vi "Teperature and FIeld Sweep_1022D.vi"() -> ()   [LabVIEW 2022 SP3]
uses:
  <vilib>/Analysis/baseanly.llb/Mean (DBL).vi
  <vilib>/Utility/file.llb/Write Delimited Spreadsheet (DBL).vi
  <vilib>/Analysis/NI_AALBase.lvlib
panel:
  in  "?":bool
  out "Temperature Status":i32(ring) items=["TemperatureUnknown"=0, "Stable"=1, "Tracking"=2, "Near"=5, "Chasing"=6, "Filling"=7, "Standby"=10, "Disabled"=13, "ImpedanceNotFunction"=14, "TempFailure"=15]
  out "Field Status":i32(ring) items=["MagnetUnknown"=0, "StablePersistent"=1, "WarmingSwitch"=2, "CoolingSwitch"=3, "StableDriven"=4, "Iterating"=5, "Charging"=6, "Discharging"=7, "CurrentError"=8, "MagnetFailure"=15]
  out "Field":dbl
  out "Temperature":dbl
  in  "Initialize":bool
  in  "System Stablization (s)":dbl=0.1 format="%#_13g"
  in  "Low Value (Oe)":dbl=-30000.0
  in  "High Value (Oe)":dbl=30000.0
  in  "Sweep Field Approach":i32(ring) items=["Linear", "NoOvershoot", "Oscillate"]
  in  "Sweep F Rate (Oe/s)":dbl=200.0 format="%#_13g"
  in  "Sweep F mode":i32(ring) items=["Persistent", "Driven"]
  in  "Set Fixed T":dbl=2.0
  in  "Fixed Temperature Approach":i32(ring)=1 items=["FastSettle", "NoOvershoot"]
  in  "FIxed T  Rate (K/min)":dbl=20.0
  out "PhaseA-F":cluster{dbl[], dbl[]}(graph)
  out "RA-F":cluster{dbl[], dbl[]}(graph)
  out "Phaseh1B-F":cluster{dbl[], dbl[]}(graph)
  out "Rh1B-F":cluster{dbl[], dbl[]}(graph)
  out "phase B 2":dbl
  in  "Phase B 2":u16(ring)=3 items=["X", "Y", "R", "Theta", "Frequency", "Noise", "Xh1", "Yh1", "Rh1", "Theta h1", "Xh2", "Yh2", "Rh2", "Theta h2"]
  out "phase A 2":dbl
  in  "Phase A 2":u16(ring)=3 items=["X", "Y", "R", "Theta", "Frequency", "Noise", "Xh1", "Yh1", "Rh1", "Theta h1", "Xh2", "Yh2", "Rh2", "Theta h2"]
  out "para1 Measurement (mV) 2":dbl=1.49013e-07
  in  "F Clear Plot A":bool
  in  "Parameter A 2":u16(ring)=2 items=["X", "Y", "R", "Theta", "Frequency", "Noise", "Xh1", "Yh1", "Rh1", "Theta h1", "Xh2", "Yh2", "Rh2", "Theta h2"]
  out "para2 Measurement (uV) 2":dbl=1.49013e-07
  in  "F Clear Plot B":bool
  in  "Parameter B 2":u16(ring)=2 items=["X", "Y", "R", "Theta", "Frequency", "Noise", "Xh1", "Yh1", "Rh1", "Theta h1", "Xh2", "Yh2", "Rh2", "Theta h2"]
  out "Field Setting":dbl format="%#_13g"
  out "Fixed Temperature":dbl
  out "Measured Field":dbl
  out "Field Status":i32(ring) items=["MagnetUnknown"=0, "StablePersistent"=1, "WarmingSwitch"=2, "CoolingSwitch"=3, "StableDriven"=4, "Iterating"=5, "Charging"=6, "Discharging"=7, "CurrentError"=8, "MagnetFailure"=15]
  out "Temperature Status":i32(ring) items=["TemperatureUnknown"=0, "Stable"=1, "Tracking"=2, "Near"=5, "Chasing"=6, "Filling"=7, "Standby"=10, "Disabled"=13, "ImpedanceNotFunction"=14, "TempFailure"=15]
  out "Measuring F":bool
  in  "Step(Oe)":i32=2000
  out "F loop run":i32
  out "Temperature Status":i32(ring) items=["TemperatureUnknown"=0, "Stable"=1, "Tracking"=2, "Near"=5, "Chasing"=6, "Filling"=7, "Standby"=10, "Disabled"=13, "ImpedanceNotFunction"=14, "TempFailure"=15]
  out "Field Status":i32(ring) items=["MagnetUnknown"=0, "StablePersistent"=1, "WarmingSwitch"=2, "CoolingSwitch"=3, "StableDriven"=4, "Iterating"=5, "Charging"=6, "Discharging"=7, "CurrentError"=8, "MagnetFailure"=15]
  out "Fixed Field":dbl
  out "Measured Temperature":dbl
  in  "Delay(T/F)":dbl=3000.0
  in  "Set FIxed F (Oe)":dbl format="%#_13g"
  in  "Fixed Field Approach":i32(ring) items=["Linear", "NoOvershoot", "Oscillate"]
  in  "FIxed F Rate (Oe/s)":dbl=100.0 format="%#_13g"
  in  "Fixed F mode":i32(ring) items=["Persistent", "Driven"]
  in  "Sweep Temperature Approach":i32(ring)=1 items=["FastSettle", "NoOvershoot"]
  in  "Sweep T  Rate (K/min)":dbl=10.0
  in  "Sweep T/F":bool=TRUE
  in  "Remote":bool=TRUE
  in  "IP Address":string="169.254.170.239"
  out "Measuring T":bool
  in  "A Sine Output Amplitude (V)":sgl=0.1
  in  "path (folder + filename)":string="G:\\My Drive\\Opticool\\Measurement\\TF dependence\\TaI23_A67_B68_267Hz_20kOhm_0.1V"
  in  "LOCKIN address":refnum<visa-resource-name>="COM4"
  out "PhaseA-T":cluster{dbl[], dbl[]}(graph)
  out "RA-T":cluster{dbl[], dbl[]}(graph)
  out "Phaseh1-T":cluster{dbl[], dbl[]}(graph)
  out "Rh1B-T":cluster{dbl[], dbl[]}(graph)
  out "phase B":dbl
  in  "Phase B":u16(ring)=9 items=["X", "Y", "R", "Theta", "Frequency", "Noise", "Xh1", "Yh1", "Rh1", "Theta h1", "Xh2", "Yh2", "Rh2", "Theta h2"]
  out "phase A":dbl
  in  "Phase A":u16(ring)=3 items=["X", "Y", "R", "Theta", "Frequency", "Noise", "Xh1", "Yh1", "Rh1", "Theta h1", "Xh2", "Yh2", "Rh2", "Theta h2"]
  out "para1 Measurement (mV)":dbl=1.49013e-07
  in  "T Clear Plot A":bool
  in  "Parameter A":u16(ring)=2 items=["X", "Y", "R", "Theta", "Frequency", "Noise", "Xh1", "Yh1", "Rh1", "Theta h1", "Xh2", "Yh2", "Rh2", "Theta h2"]
  out "para2 Measurement (uV)":dbl=1.49013e-07
  in  "T Clear Plot B":bool
  in  "Parameter B":u16(ring)=8 items=["X", "Y", "R", "Theta", "Frequency", "Noise", "Xh1", "Yh1", "Rh1", "Theta h1", "Xh2", "Yh2", "Rh2", "Theta h2"]
  out "Temperature Setting":dbl format="%#_13g"
  in  "Save data or not":bool=TRUE
  in  "Step(K)":i32=10
  out "T loop run":i32
  in  "B frequency":dbl=267.7 format="%#_13g"
  in  "B Input Connection (0: Single-Ended)":u16(ring)=1 items=["Single-Ended Voltage", "Differential Voltage", "1 MOhm Current Gain", "100 MOhm Current Gain"]
  in  "B harmonic 1":u8=2
  in  "B harmonic 2":u8=3
  in  "B reference Manual Phase":dbl=-59.75
  in  "auto phase B":bool=TRUE
  in  "B Sample time (s)":dbl=0.001 min=0.001 max=100.0 step=0.001
  in  "B Sensitivity":u16(ring)=20 items=["1 nV/fA", "2 nV/fA", "5 nV/fA", "10 nV/fA", "20 nV/fA", "50 nV/fA", "100 nV/fA", "200 nV/fA", "500 nV/fA", "1 uV/pA", "2 uV/pA", "5 uV/pA", "10 uV/pA", "20 uV/pA", "50 uV/pA", "100 uV/pA", "200 uV/pA", "500 uV/pA", "1 mV/nA", "2 mV/nA", "5 mV/nA", "10 mV/nA", "20 mV/nA", "50 mV/nA", "100 mV/nA", "200 mV/nA", "500 mV/nA", "1 V/uA"]
  in  "Enable Sync Filter B (open when f<200Hz)":bool
  in  "B Time Constant":u8(ring)=9 items=["10 us", "30 us", "100 us", "300 us", "1 ms", "3 ms", "10 ms", "30 ms", "100 ms", "300 ms", "1 s", "3 s", "10 s", "30 s", "100 s", "300 s", "1 ks", "3 ks"]
  in  "B Reference Source":u8(ring)=3 items=["External", "Internal", "Internal Sweep", "Channel-A"]
  in  "B Low Pass Filter Slope":u8(ring)=2 items=["6 dB/oct", "12 dB/oct", "18 db/oct", "24 dB/oct"]
  in  "A frequency":dbl=267.7 format="%#_13g"
  in  "A Input Connection (0: Single-Ended)":u16(ring)=1 items=["Single-Ended Voltage", "Differential Voltage", "1 MOhm Current Gain", "100 MOhm Current Gain"]
  in  "A harmonic 1":u8=2
  in  "A harmonic 2":u8=3
  in  "A reference Manual Phase":dbl=-59.75
  in  "auto phase A":bool=TRUE
  in  "A Reference Source":u8(ring)=1 items=["External", "Internal", "Internal Sweep"]
  in  "A Sample time (s)":dbl=0.001 min=0.001 max=100.0 step=0.001
  in  "A Time Constant":u8(ring)=9 items=["10 us", "30 us", "100 us", "300 us", "1 ms", "3 ms", "10 ms", "30 ms", "100 ms", "300 ms", "1 s", "3 s", "10 s", "30 s", "100 s", "300 s", "1 ks", "3 ks"]
  in  "Enable Sync Filter A (open when f<200Hz)":bool
  in  "A Sensitivity":u16(ring)=20 items=["1 nV/fA", "2 nV/fA", "5 nV/fA", "10 nV/fA", "20 nV/fA", "50 nV/fA", "100 nV/fA", "200 nV/fA", "500 nV/fA", "1 uV/pA", "2 uV/pA", "5 uV/pA", "10 uV/pA", "20 uV/pA", "50 uV/pA", "100 uV/pA", "200 uV/pA", "500 uV/pA", "1 mV/nA", "2 mV/nA", "5 mV/nA", "10 mV/nA", "20 mV/nA", "50 mV/nA", "100 mV/nA", "200 mV/nA", "500 mV/nA", "1 V/uA"]
  in  "A Low Pass Filter Slope":u8(ring)=2 items=["6 dB/oct", "12 dB/oct", "18 db/oct", "24 dB/oct"]
  in  "stabilization(S)":dbl=0.1 format="%#_13g"
  in  "High Value (K)":dbl=300.0
  in  "Low Value (K)":dbl=2.0
  in  "loop #":i32=1
  # "Statue"
  # "Lock-in Setting"
  # "Channel A"
  # "Channel B"
  # "Sweep F Mesurement"
  # "Temprature and Field Setting"
  # "Sweep T Mesurement"
  # "Sweep F"
  # "Sweep T"
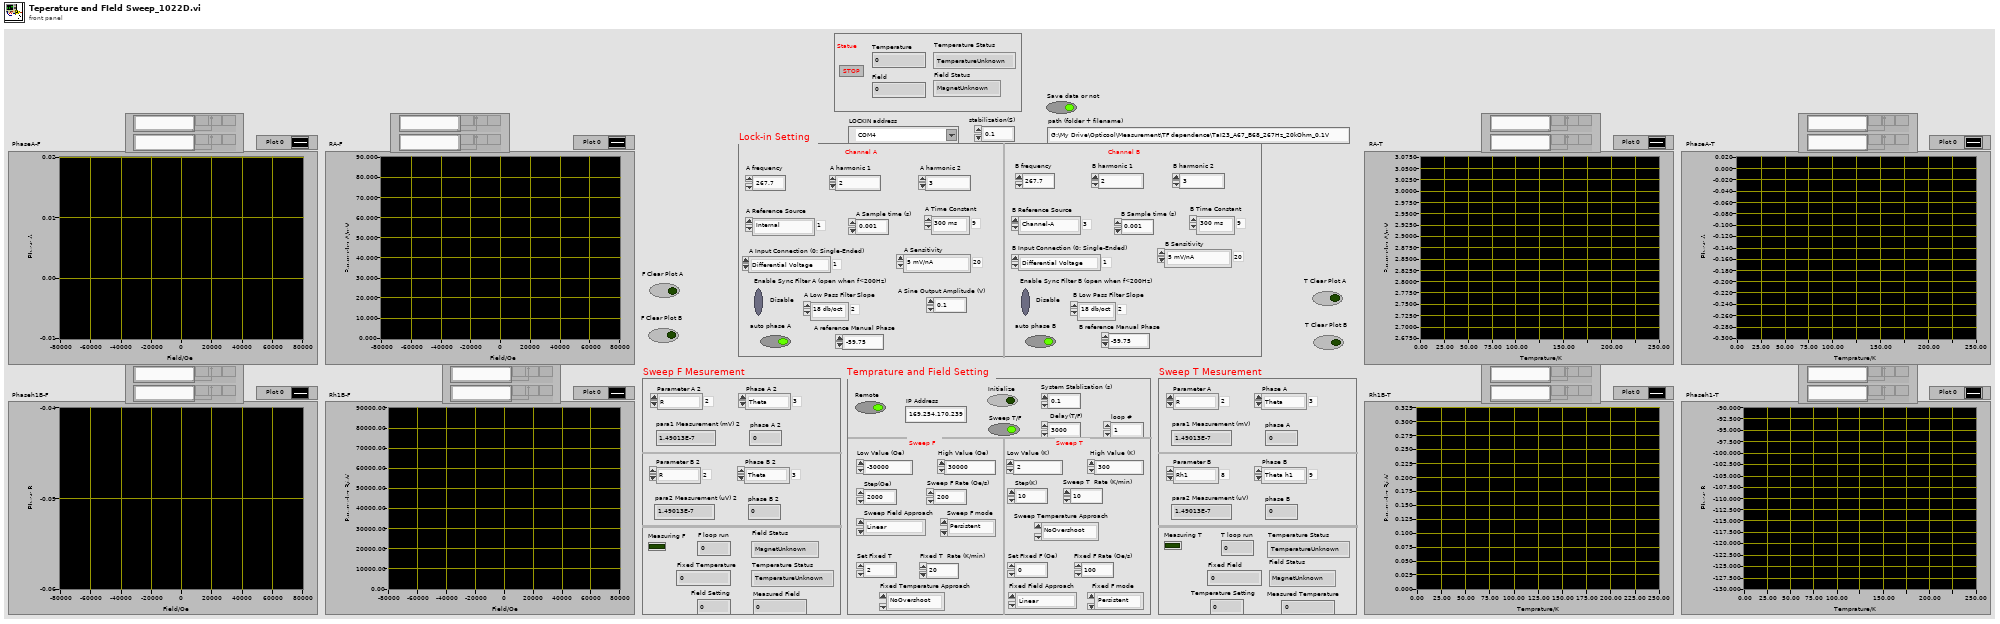
[diagram p1: front panel]
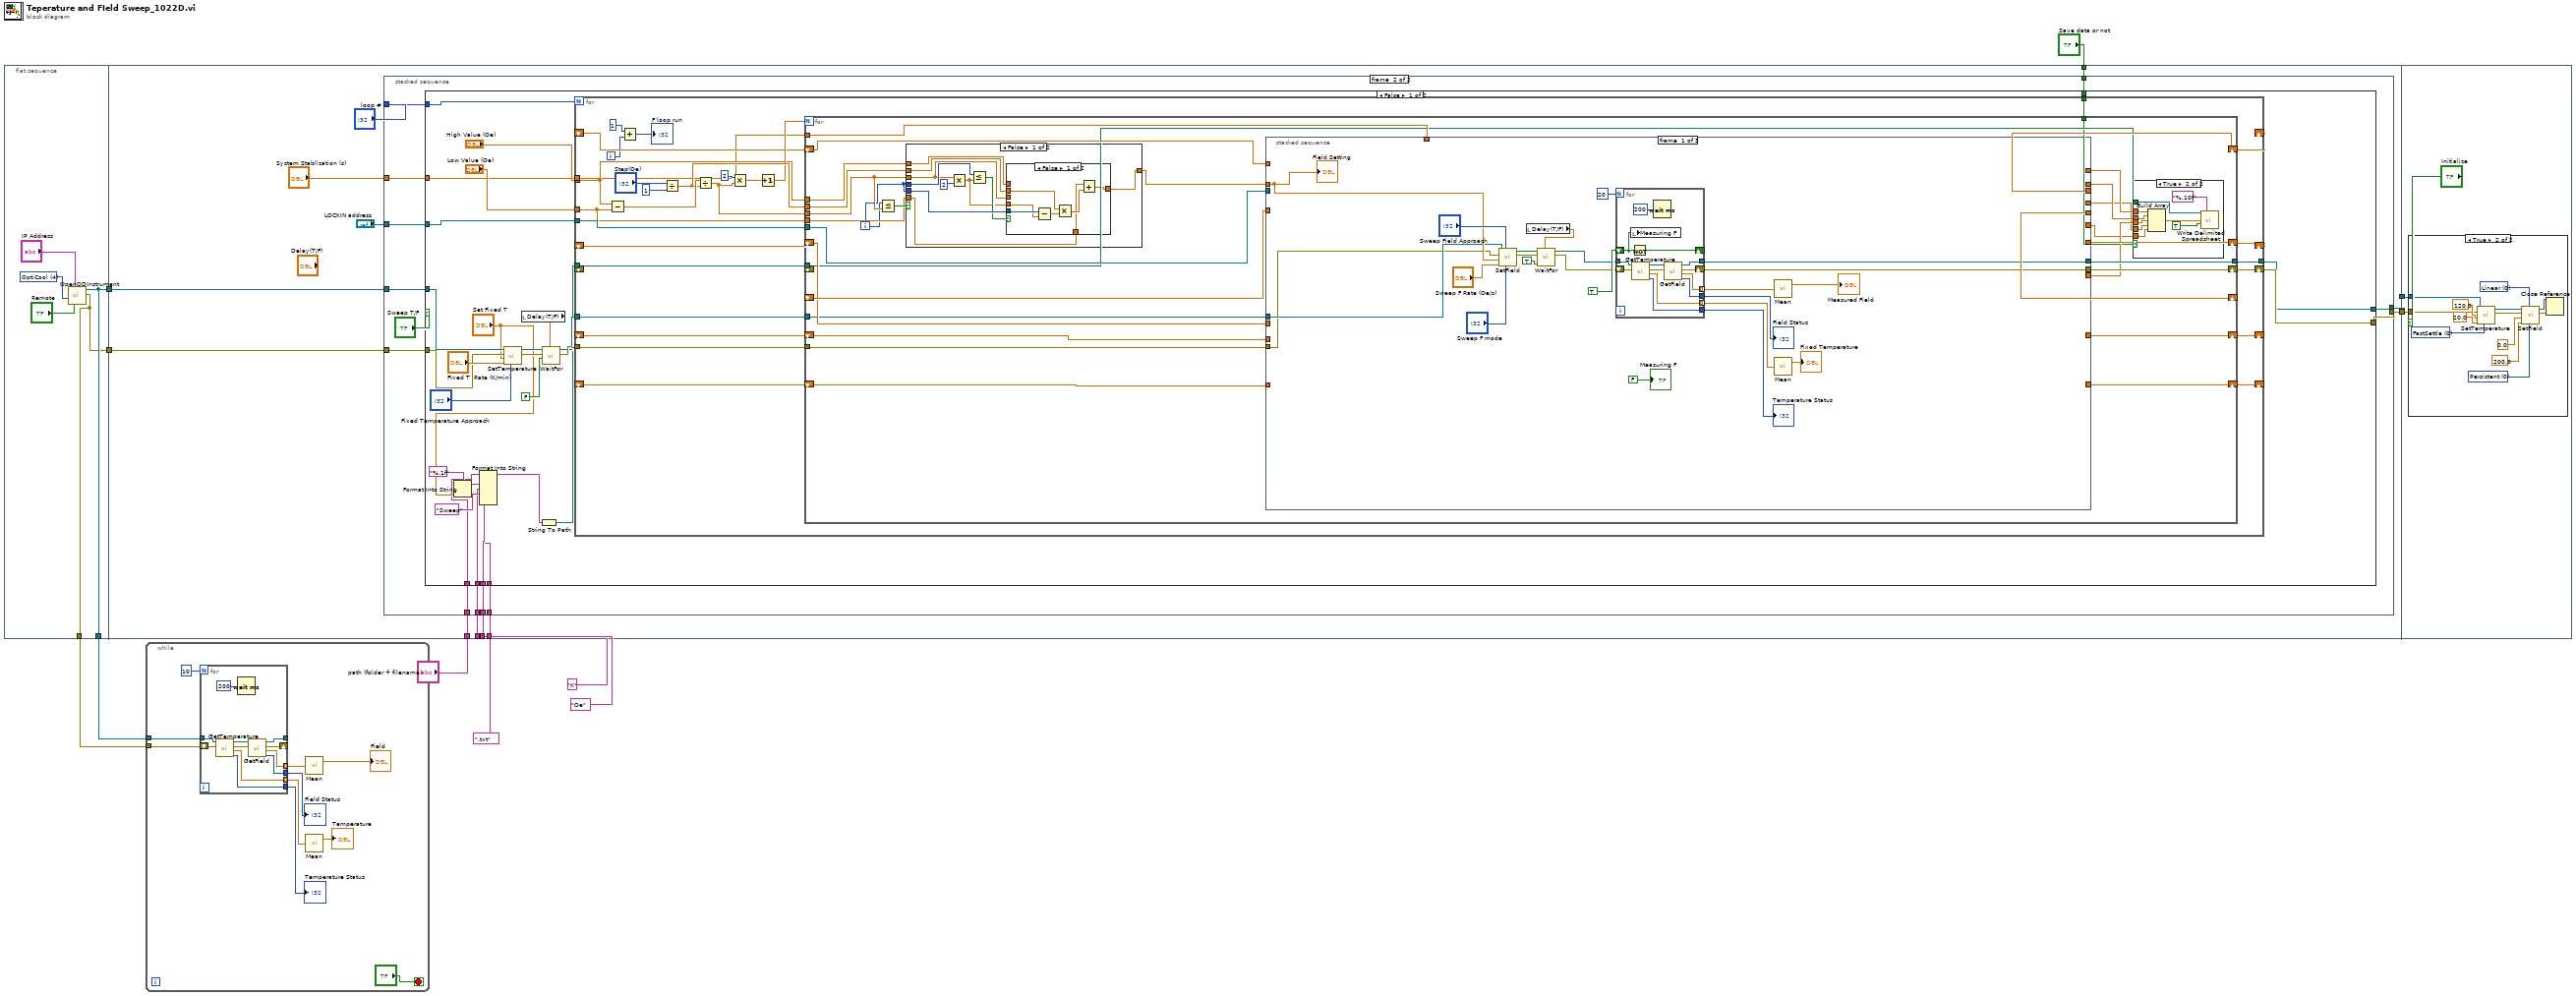
[diagram p0: block diagram]
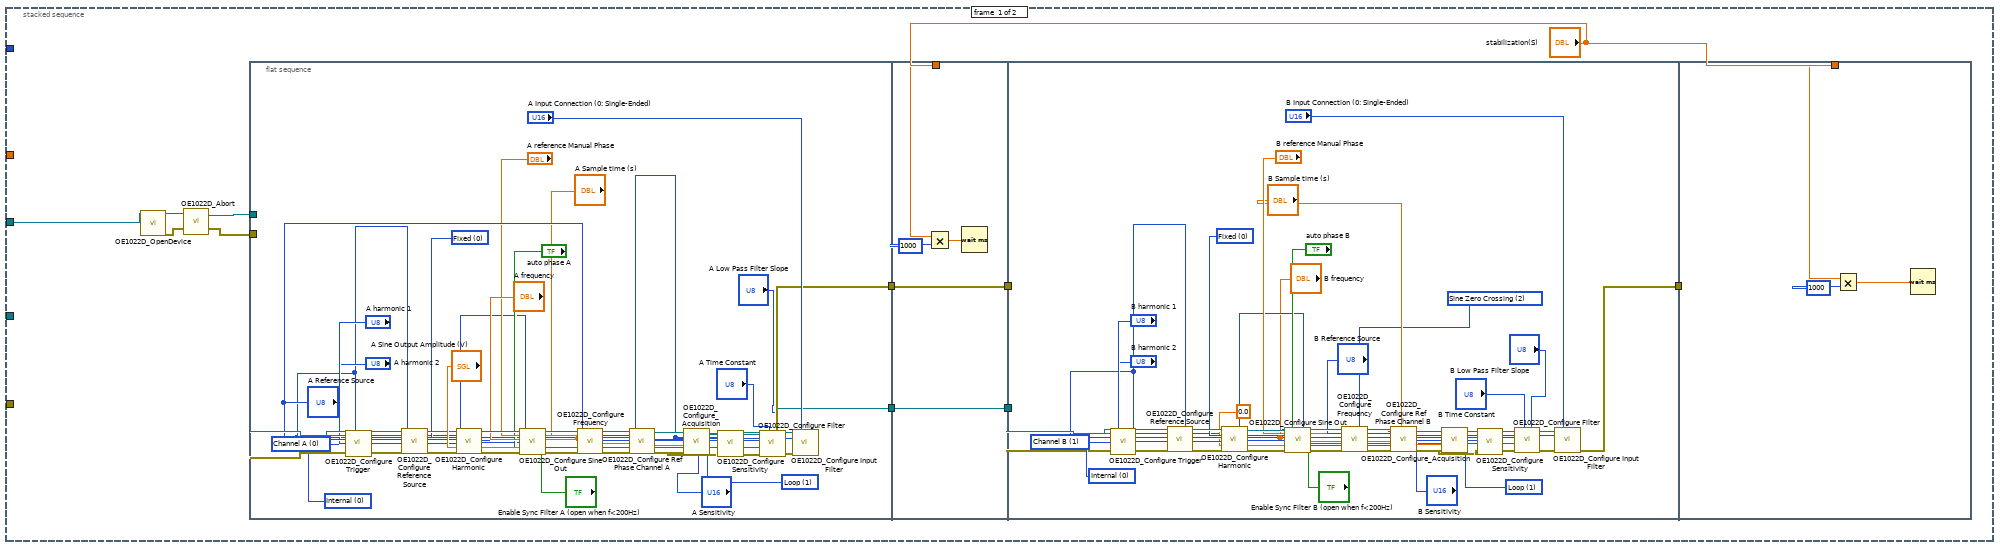
[diagram p2: hidden frame]
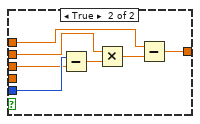
[diagram p4: hidden frame]
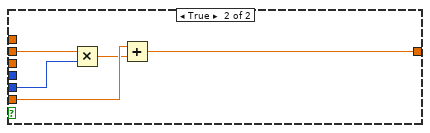
[diagram p5: hidden frame]
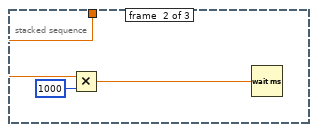
[diagram p6: hidden frame]
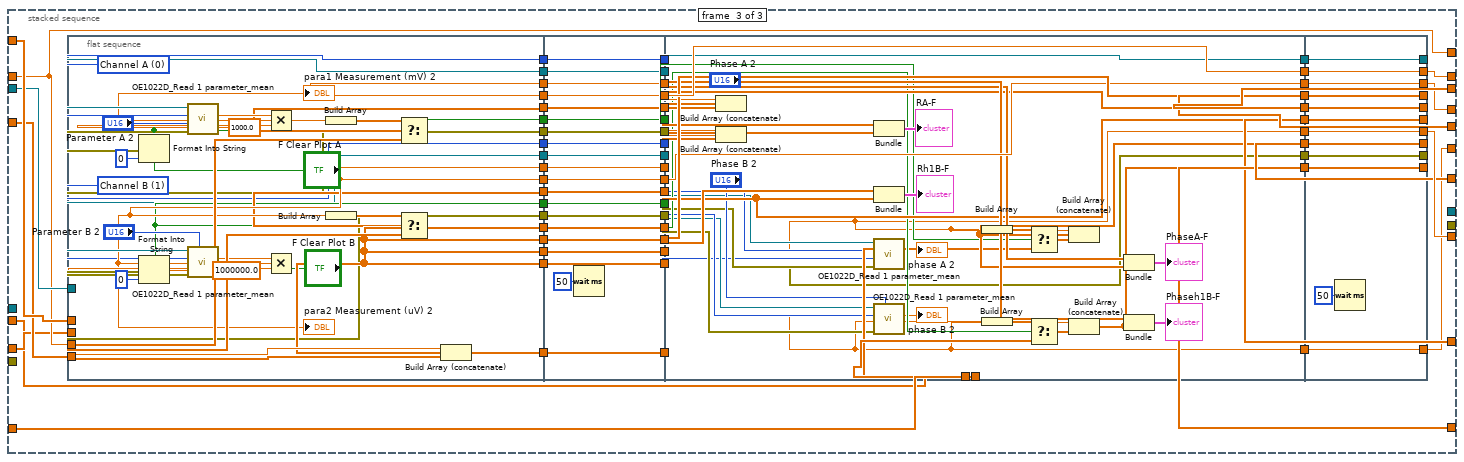
[diagram p7: hidden frame]
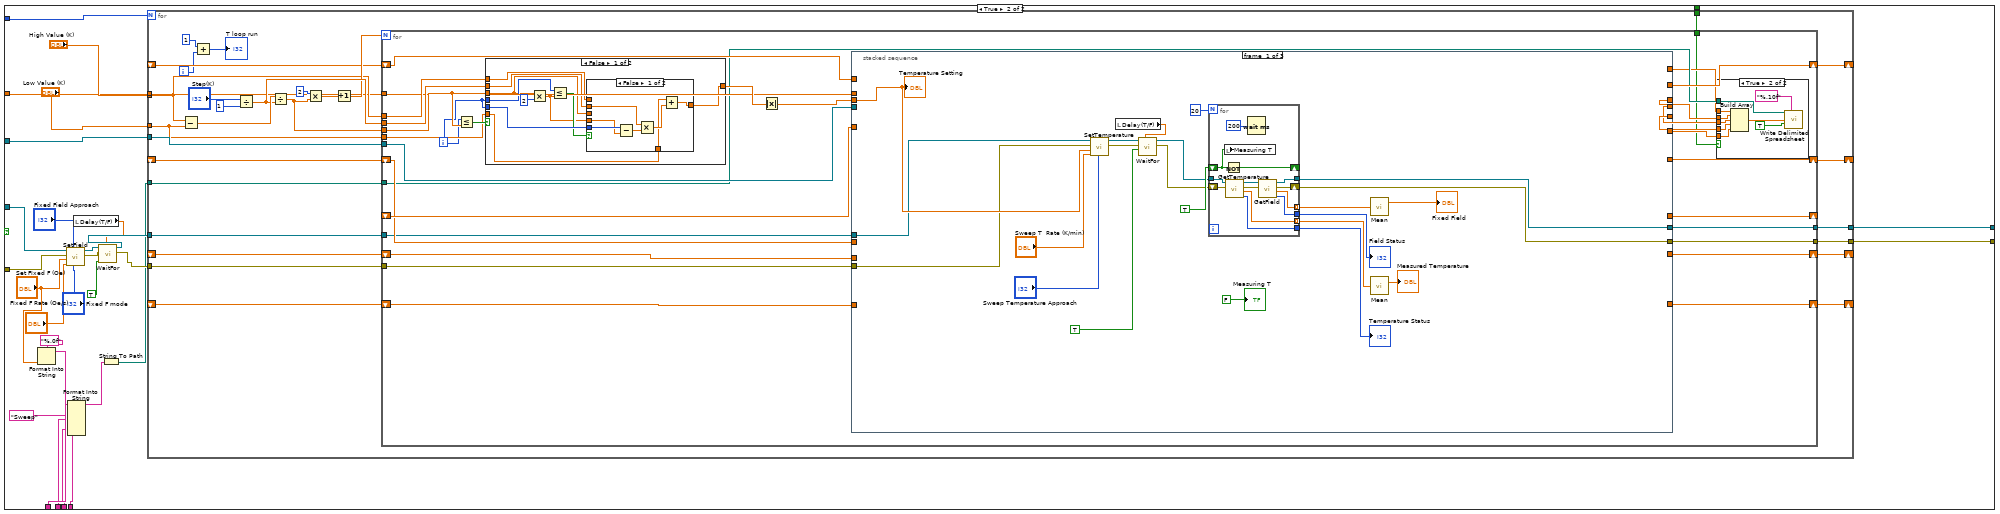
[diagram p8: hidden frame]
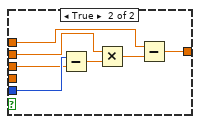
[diagram p10: hidden frame]
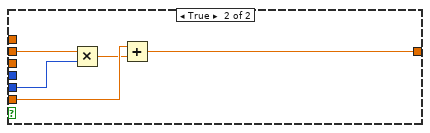
[diagram p11: hidden frame]
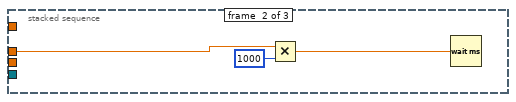
[diagram p12: hidden frame]
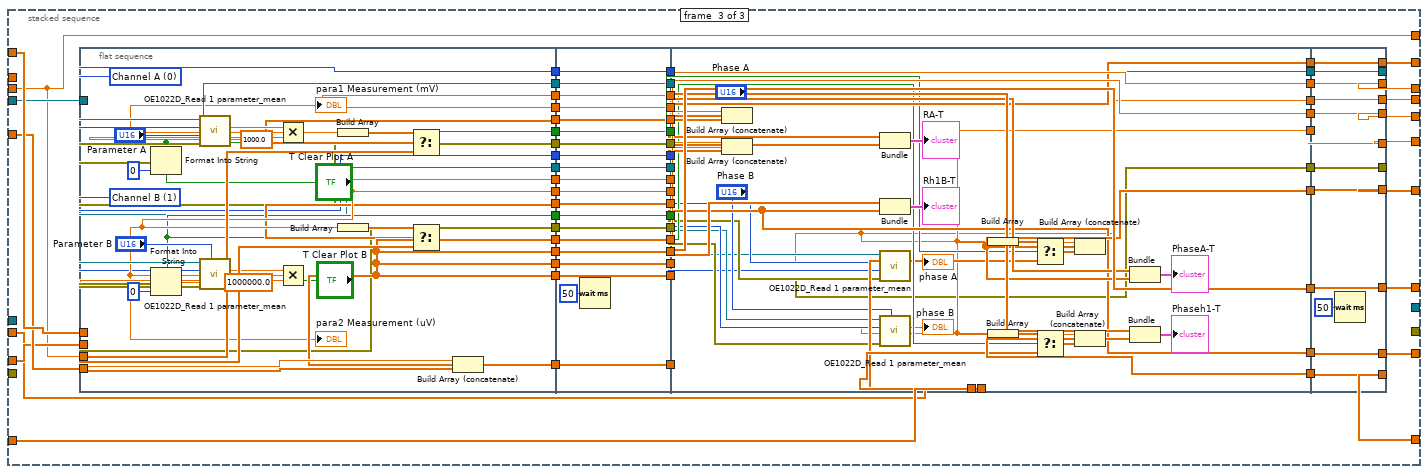
[diagram p13: hidden frame]
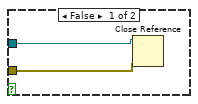
[diagram p14: hidden frame]
diagram:
  n1 = flat-sequence {
    tunnel: [w13] -> w11
    tunnel: [w12] -> w10
    tunnel: [w13] -> w3
    tunnel: [w12] -> w2
    tunnel: w11 -> [w26]
    tunnel: w10 -> [w25]
    tunnel: "path (folder + filename)" -> [w24]
    tunnel: "Oe" -> [w23]
    tunnel: "K" -> [w22]
    tunnel: ".txt" -> [w21]
    tunnel: [w19] -> w5
    tunnel: [w18] -> w4
    tunnel: "Save data or not" -> [w17]
    tunnel: w5 -> [w800]
    tunnel: w4 -> [w799]
    frame #0 {
      w14 = 4 items=["PPMS", "VersaLab", "DynaCool", "SVSM", "OptiCool"] ("InstrumentType")
      n2 = call "OpenQDInstrument.vi"("Remote"="Remote", "IP Address"="IP Address", "InstrumentType"=w14) -> ("error out"=w12:errorcluster, "Instrument Ref"=w13:refnum<k24>)  [unwired: 5 in]
    }
    frame #1 {
      n3 = stacked-sequence {
        tunnel: "LOCKIN address" -> [w31 w138]
        tunnel: "loop #" -> [_ w137]
        tunnel: w26 -> [_ w135]
        tunnel: w25 -> [_ w134]
        tunnel: w24 -> [_ w133]
        tunnel: w23 -> [_ w132]
        tunnel: w22 -> [_ w131]
        tunnel: w21 -> [_ w130]
        tunnel: "System Stablization (s)" -> [_ w129]
        tunnel: [_ w128] -> w19
        tunnel: [_ w127] -> w18
        tunnel: w17 -> [_ w126]
        frame #0 {
          n4 = call <instrlib>:"OE1022D_OpenDevice.vi"("VISA resource name"=w31) -> ("VISA资源名称输出"=w30:refnum<visa-resource-name>, "错误输出"=w32:errorcluster)  [unwired: 17 in]
          n5 = call <instrlib>:"OE1022D_Abort.vi"("error in (no error)"=w32, "VISA resource name"=w30) -> ("error out"=w37:errorcluster, "VISA resource name out"=w38:refnum<visa-resource-name>)
          n6 = flat-sequence {
            tunnel: w38 -> [w78]
            tunnel: [w66] -> w36
            tunnel: w37 -> [w77]
            tunnel: [w54] -> w34
            tunnel: w36 -> [w83]
            tunnel: [w83] -> w35
            tunnel: w34 -> [w82]
            tunnel: [w82] -> w33
            tunnel: "stabilization(S)" -> [w79]
            tunnel: w35 -> [w105]
            tunnel: [w104] -> w39
            tunnel: w33 -> [w103]
            tunnel: w39 -> [_]
            tunnel: "stabilization(S)" -> [w123]
            frame #0 {
              w40 = u8 1 items=["Single", "Loop"] ("Sample Mode (Single/Loop)")
              w53 = u8 0 items=["Fixed", "Linear", "Log"] ("SineOut Mode")
              w55 = u16 0 items=["Internal", "External"] ("Trigger Source (0: Internal)")
              w44 = u8 0 items=["Channel A", "Channel B"] ("OE1022D A/B")
              n7 = call <instrlib>:"OE1022D_Configure Trigger.vi"("Trigger Source (0: Internal)"=w55, "error in (no error)   2"=w77, "OE1022D A/B"=w44, "VISA resource name   2"=w78) -> ("error out   2"=w71:errorcluster, "VISA resource name out   2"=w72:refnum<visa-resource-name>)
              n8 = call <instrlib>:"OE1022D_Configure Reference Source.vi"("VISA resource name"=w72, "OE1022D A/B"=w44, "Reference Source"="A Reference Source", "error in (no error)"=w71) -> ("VISA resource name out"=w70:refnum<visa-resource-name>, "error out"=w68:errorcluster)  [unwired: 14 in]
              n9 = call <instrlib>:"OE1022D_Configure Harmonic.vi"("VISA resource name"=w70, "OE1022D A/B"=w44, "Harmonic 1"="A harmonic 1", "Harmonic 2"="A harmonic 2", "error in (no error)"=w68) -> ("VISA resource name out"=w69:refnum<visa-resource-name>, "error out"=w67:errorcluster)  [unwired: 13 in]
              n10 = call <instrlib>:"OE1022D_Configure Sine Out.vi"("VISA resource name"=w69, "SineOut Mode"=w53, "OE1022D A/B"=w44, "Sine Output Amplitude (V)"="A Sine Output Amplitude (V)", "error in (no error)"=w67) -> ("VISA resource name out"=w75:refnum<visa-resource-name>, "error out"=w74:errorcluster)  [unwired: 9 in]
              n11 = call <instrlib>:"OE1022D_Configure Frequency.vi"("VISA resource name"=w75, "OE1022D A/B"=w44, "Internal Frequency(Hz)"="A frequency", "error in (no error)"=w74) -> ("VISA resource name out"=w65:refnum<visa-resource-name>, "error out"=w62:errorcluster)  [unwired: 14 in]
              n12 = call <instrlib>:"OE1022D_Configure Ref Phase Channel A.vi"("VISA resource name"=w65, "Reference Source"="A Reference Source", "Internal Frequency(Hz)"="A frequency", "Auto Phase (T: Enabled)"="auto phase A", "error in (no error)"=w62, "Manual Phase  (degree)"="A reference Manual Phase") -> ("VISA resource name out"=w64:refnum<visa-resource-name>, "error out"=w63:errorcluster)  [unwired: 12 in]
              n13 = call <instrlib>:"OE1022D_Configure_Acquisition.vi"("VISA resource name"=w64, "OE1022D A/B"=w44, "Sample time (s)"="A Sample time (s)", "error in (no error)"=w63, "Sample Mode (Single/Loop)"=w40) -> ("VISA resource name out"=w47:refnum<visa-resource-name>, "error out"=w46:errorcluster)  [unwired: 3 in]
              n14 = call <instrlib>:"OE1022D_Configure Sensitivity.vi"("VISA resource name"=w47, "OE1022D A/B"=w44, "Sensitivity"="A Sensitivity", "error in (no error)"=w46) -> ("VISA resource name out"=w51:refnum<visa-resource-name>, "error out"=w50:errorcluster)  [unwired: 14 in]
              n15 = call <instrlib>:"OE1022D_Configure Filter.vi"("Low Pass Filter Slope (1: 12dB/oct)"="A Low Pass Filter Slope", "Time Constant (8: 100ms)"="A Time Constant", "error in (no error)"=w50, "Enable Sync Filter (F: Disable)"="Enable Sync Filter A (open when f<200Hz)", "OE1022D A/B"=w44, "VISA resource name"=w51) -> ("error out"=w48:errorcluster, "VISA resource name out"=w49:refnum<visa-resource-name>)  [unwired: 4 in]
              n16 = call <instrlib>:"OE1022D_Configure Input Filter.vi"("VISA resource name"=w49, "Input Source"="A Input Connection (0: Single-Ended)", "OE1022D A/B"=w44, "error in (no error)"=w48) -> ("VISA resource name out"=w54:refnum<visa-resource-name>, "error out"=w66:errorcluster)  [unwired: 10 in]
            }
            frame #1 {
              n17 = Multiply(x=w79, y=1000) -> (x*y=w81:dbl)
              n18 = Wait (ms)(milliseconds to wait=w81) -> ()  [unwired: 1 out]
            }
            frame #2 {
              w85 = u8 1 items=["Single", "Loop"] ("Sample Mode (Single/Loop)")
              w87 = u8 2 items=["TTL Pos", "TTL Neg", "Sine Zero Crossing"] ("External Ref Trigger")
              w100 = u8 0 items=["Fixed", "Linear", "Log"] ("SineOut Mode")
              w106 = u16 0 items=["Internal", "External"] ("Trigger Source (0: Internal)")
              w92 = u8 1 items=["Channel A", "Channel B"] ("OE1022D A/B")
              n19 = call <instrlib>:"OE1022D_Configure Trigger.vi"("Trigger Source (0: Internal)"=w106, "error in (no error)   2"=w105, "OE1022D A/B"=w92, "VISA resource name   2"=w103) -> ("error out   2"=w118:errorcluster, "VISA resource name out   2"=w119:refnum<visa-resource-name>)
              n20 = call <instrlib>:"OE1022D_Configure Reference Source.vi"("VISA resource name"=w119, "OE1022D A/B"=w92, "error in (no error)"=w118) -> ("VISA resource name out"=w117:refnum<visa-resource-name>, "error out"=w115:errorcluster)  [unwired: 15 in]
              n21 = call <instrlib>:"OE1022D_Configure Harmonic.vi"("VISA resource name"=w117, "OE1022D A/B"=w92, "Harmonic 1"="B harmonic 1", "Harmonic 2"="B harmonic 2", "error in (no error)"=w115) -> ("VISA resource name out"=w116:refnum<visa-resource-name>, "error out"=w114:errorcluster)  [unwired: 13 in]
              n22 = call <instrlib>:"OE1022D_Configure Sine Out.vi"("VISA resource name"=w116, "SineOut Mode"=w100, "OE1022D A/B"=w92, "Sine Output Amplitude (V)"=sgl 0.0, "error in (no error)"=w114) -> ("VISA resource name out"=w121:refnum<visa-resource-name>, "error out"=w120:errorcluster)  [unwired: 9 in]
              n23 = call <instrlib>:"OE1022D_Configure Frequency.vi"("VISA resource name"=w121, "OE1022D A/B"=w92, "Internal Frequency(Hz)"="B frequency", "error in (no error)"=w120) -> ("VISA resource name out"=w113:refnum<visa-resource-name>, "error out"=w110:errorcluster)  [unwired: 14 in]
              n24 = call <instrlib>:"OE1022D_Configure Ref Phase Channel B.vi"("VISA resource name"=w113, "Reference Source"="B Reference Source", "External Ref Trigger"=w87, "Internal Frequency(Hz)"="B frequency", "Auto Phase (T: Enabled)"="auto phase B", "error in (no error)"=w110, "Manual Phase  (degree)"="B reference Manual Phase") -> ("VISA resource name out"=w112:refnum<visa-resource-name>, "error out"=w111:errorcluster)  [unwired: 11 in]
              n25 = call <instrlib>:"OE1022D_Configure_Acquisition.vi"("VISA resource name"=w112, "OE1022D A/B"=w92, "Sample time (s)"="B Sample time (s)", "error in (no error)"=w111, "Sample Mode (Single/Loop)"=w85) -> ("VISA resource name out"=w93:refnum<visa-resource-name>, "error out"=w94:errorcluster)  [unwired: 3 in]
              n26 = call <instrlib>:"OE1022D_Configure Sensitivity.vi"("VISA resource name"=w93, "OE1022D A/B"=w92, "Sensitivity"="B Sensitivity", "error in (no error)"=w94) -> ("VISA resource name out"=w97:refnum<visa-resource-name>, "error out"=w96:errorcluster)  [unwired: 14 in]
              n27 = call <instrlib>:"OE1022D_Configure Filter.vi"("Low Pass Filter Slope (1: 12dB/oct)"="B Low Pass Filter Slope", "Time Constant (8: 100ms)"="B Time Constant", "error in (no error)"=w96, "Enable Sync Filter (F: Disable)"="Enable Sync Filter B (open when f<200Hz)", "OE1022D A/B"=w92, "VISA resource name"=w97) -> ("error out"=w95:errorcluster, "VISA resource name out"=w84:refnum<visa-resource-name>)  [unwired: 4 in]
              n28 = call <instrlib>:"OE1022D_Configure Input Filter.vi"("VISA resource name"=w84, "Input Source"="B Input Connection (0: Single-Ended)", "OE1022D A/B"=w92, "error in (no error)"=w95) -> ("error out"=w104:errorcluster)  [unwired: 10 in, 1 out]
            }
            frame #3 {
              n29 = Multiply(x=w123, y=1000) -> (x*y=w125:dbl)
              n30 = Wait (ms)(milliseconds to wait=w125) -> ()  [unwired: 1 out]
            }
          }
        }
        frame #1 {
          n31 = case shown="False" "Sweep T/F" {
            tunnel: w138 -> [w165 w496]
            tunnel: w137 -> [w166 w495]
            tunnel: w135 -> [w158 w491]
            tunnel: w134 -> [w159 w490]
            tunnel: w133 -> [w149 w480]
            tunnel: w132 -> [w148 w476]
            tunnel: w131 -> [w147 w477]
            tunnel: w130 -> [w146 w475]
            tunnel: w129 -> [w143 w472]
            tunnel: [w142 w471] -> w128
            tunnel: [w141 w470] -> w127
            tunnel: w126 -> [w140 w469]
            frame False {
              n32 = Format Into String(format string="%.1f", "Set Fixed T") -> (resulting string=w152:string)  [unwired: 2 in, 1 out]
              n33 = Format Into String(initial string=w149, w152, w147, "Sweep", w148, w146) -> (resulting string=w153:string)  [unwired: 2 in, 1 out]
              n34 = call "SetTemperature.vi"("Approach"="Fixed Temperature Approach", "Rate"="FIxed T  Rate (K/min)", "Temperature"="Set Fixed T", "error in (no error)"=w159, "Instrument Ref In"=w158) -> ("error out"=w160:errorcluster, "Instrument Ref Out"=w161:refnum<k24>)  [unwired: 2 in, 1 out]
              n35 = local read "Delay(T/F)"() -> (w139:dbl)
              n36 = String To Path(string=w153) -> (path=w150:path)
              n37 = call "WaitFor.vi"("Delay"=w139, "Wait For Temperature"=FALSE ("WaitForTemperature"), "error in (no error)"=w160, "Instrument Ref In"=w161) -> ("error out"=w157:errorcluster, "Instrument Ref Out"=w156:refnum<k24>)  [unwired: 6 in]
              n38 = for {
                N: w166 -> [_]
                tunnel: w165 -> [w195]
                tunnel: "Low Value (Oe)" -> [w189]
                tunnel: "High Value (Oe)" -> [w179]
                tunnel: w150 -> [w188]
                shift-right: [w184] -> _
                shift-left: _ -> [w183]
                shift-right: [w178] -> _
                shift-left: _ -> [w177]
                shift-right: [w176] -> _
                shift-left: _ -> [w175]
                shift-right: [w174] -> _
                shift-left: _ -> [w173]
                tunnel: w156 -> [w172]
                tunnel: w157 -> [w171]
                tunnel: w143 -> [w170]
                shift-right: [w169] -> w142
                shift-left: _ -> [_]
                tunnel: [w168] -> w141
                tunnel: w140 -> [w167]
                i -> [w181]
                n39 = Subtract(x=w179, y=w189) -> (x-y=w191:dbl)
                n40 = Add(x=1, y=w181) -> (x+y=→"F loop run":i32)
                n41 = Divide(x="Step(Oe)", y=1) -> (x/y=w190:dbl)
                n42 = Divide(x=w191, y=w190) -> (x/y=w187:dbl)
                n43 = Multiply(x=2, y=w187) -> (x*y=w186:dbl)
                n44 = Increment(x=w186) -> (x+1=w185:dbl)
                n45 = for {
                  N: w185 -> [_]
                  tunnel: w195 -> [w225]
                  tunnel: w190 -> [w221]
                  shift-right: [w213] -> w184
                  shift-left: w183 -> [w224]
                  tunnel: w187 -> [w219]
                  tunnel: w189 -> [w222]
                  tunnel: w179 -> [w220]
                  tunnel: w188 -> [w202]
                  shift-right: [w212] -> _
                  shift-left: _ -> [w216]
                  shift-right: [w215] -> w178
                  shift-left: w177 -> [w214]
                  shift-right: [w211] -> w176
                  shift-left: w175 -> [w210]
                  shift-right: [w209] -> w174
                  shift-left: w173 -> [w208]
                  tunnel: w172 -> [w207]
                  tunnel: w171 -> [w206]
                  tunnel: w170 -> [w205]
                  shift-right: [w204] -> w169
                  shift-left: _ -> [_]
                  tunnel: [w203] -> w168
                  tunnel: w167 -> [w196]
                  i -> [w218]
                  n46 = Less Or Equal?(x=w218, y=w219) -> (x <= y?=w223:bool)
                  n47 = case shown="False" w223 {
                    tunnel: w222 -> [w235 w263]
                    tunnel: w218 -> [w244 w262]
                    tunnel: w221 -> [w243 w261]
                    tunnel: [w241 w259] -> w217
                    tunnel: w220 -> [w242 _]
                    tunnel: w219 -> [w237 _]
                    tunnel: w218 -> [w240 _]
                    frame False {
                      n48 = Multiply(x=w237, y=2) -> (x*y=w236:dbl)
                      n49 = Less Or Equal?(x=w240, y=w236) -> (x <= y?=w238:bool)
                      n50 = case shown="False" w238 {
                        tunnel: w244 -> [w251 w258]
                        tunnel: w243 -> [w249 w256]
                        tunnel: w242 -> [_ w254]
                        tunnel: [w247 w253] -> w241
                        tunnel: w237 -> [_ w252]
                        tunnel: w236 -> [w246 _]
                        tunnel: w235 -> [w245 _]
                        frame False {
                          n51 = Subtract(x=w251, y=w246) -> (x-y=w250:dbl)
                          n52 = Multiply(x=w249, y=w250) -> (x*y=w248:dbl)
                          n53 = Add(x=w245, y=w248) -> (x+y=w247:dbl)
                        }
                        frame True {
                          n54 = Subtract(x=w258, y=w252) -> (x-y=w257:dbl)
                          n55 = Multiply(x=w256, y=w257) -> (x*y=w255:dbl)
                          n56 = Subtract(x=w254, y=w255) -> (x-y=w253:dbl)
                        }
                      }
                    }
                    frame True {
                      n57 = Multiply(x=w261, y=w262) -> (x*y=w260:dbl)
                      n58 = Add(x=w263, y=w260) -> (x+y=w259:dbl)
                    }
                  }
                  n59 = stacked-sequence {
                    tunnel: w225 -> [_ _ w365]
                    tunnel: w217 -> [w269 _ w364]
                    tunnel: w224 -> [_ _ w367]
                    tunnel: [_ _ w366] -> w213
                    tunnel: [_ _ w303] -> w200
                    tunnel: [_ _ w364] -> w201
                    tunnel: [_ _ w363] -> w212
                    tunnel: w216 -> [_ _ w362]
                    tunnel: [_ _ w361] -> w199
                    tunnel: [_ _ w360] -> w215
                    tunnel: w214 -> [_ _ w353]
                    tunnel: [_ _ w359] -> w211
                    tunnel: w210 -> [_ _ w354]
                    tunnel: [_ _ w358] -> w209
                    tunnel: w208 -> [_ _ w357]
                    tunnel: [_ _ w356] -> w197
                    tunnel: [_ _ w355] -> w198
                    tunnel: w207 -> [w268 _ _]
                    tunnel: w206 -> [w267 _ _]
                    tunnel: w205 -> [_ w300 _]
                    tunnel: [w266 _ _] -> w204
                    tunnel: [w265 _ _] -> w203
                    frame #0 {
                      n60 = call "SetField.vi"("Mode"="Sweep F mode", "Approach"="Sweep Field Approach", "Rate"="Sweep F Rate (Oe/s)", "Field"=w269, "error in (no error)"=w267, "Instrument Ref In"=w268) -> ("error out"=w273:errorcluster, "Instrument Ref Out"=w274:refnum<k24>)  [unwired: 1 in, 1 out]
                      n61 = local read "Delay(T/F)"() -> (w264:dbl)
                      n62 = call "WaitFor.vi"("Delay"=w264, "Wait For Field"=TRUE, "error in (no error)"=w273, "Instrument Ref In"=w274) -> ("error out"=w271:errorcluster, "Instrument Ref Out"=w270:refnum<k24>)  [unwired: 6 in]
                      n63 = for {
                        N: 20 -> [_]
                        shift-right: [w299] -> _
                        shift-left: TRUE -> [w297]
                        shift-right: [w294] -> w266
                        shift-left: w271 -> [w296]
                        tunnel: w270 -> [w293]
                        tunnel: [w291] -> w265
                        tunnel: [w288] -> w284
                        tunnel: [w287] -> w283
                        tunnel: [w289] -> w281 mode=indexing
                        tunnel: [w290] -> w282 mode=indexing
                        n64 = local write "Measuring F"(w297) -> ()
                        n65 = Not(x=w297) -> (.not. x?=w299:bool)
                        n66 = call "GetTemperature.vi"("error in (no error)"=w296, "Instrument Ref In"=w293) -> ("Temperature\nStatus"=w287:i32, "Temperature"=w290:dbl, "error out"=w295:errorcluster, "Instrument Ref Out"=w292:refnum<k24>)  [unwired: 3 in, 1 out]
                        n67 = Wait (ms)(milliseconds to wait=u32 200) -> ()  [unwired: 1 out]
                        n68 = call "GetField.vi"("error in (no error)"=w295, "Instrument Ref In"=w292) -> ("Field\nStatus"=w288:i32, "Field"=w289:dbl, "error out"=w294:errorcluster, "Instrument Ref Out"=w291:refnum<k24>)  [unwired: 3 in, 1 out]
                      }
                      "Field Status" <- w284
                      "Temperature Status" <- w283
                      n69 = call-poly <vilib>:"Mean.vi"("X"=w281) -> ("mean"=→"Measured Field":dbl)  [unwired: 1 out]
                      n70 = call-poly <vilib>:"Mean.vi"("X"=w282) -> ("mean"=→"Fixed Temperature":dbl)  [unwired: 1 out]
                      "Field Setting" <- w269
                      "Measuring F" <- FALSE
                    }
                    frame #1 {
                      n71 = Multiply(x=w300, y=1000) -> (x*y=w302:dbl)
                      n72 = Wait (ms)(milliseconds to wait=w302) -> ()  [unwired: 1 out]
                    }
                    frame #2 {
                      n73 = flat-sequence {
                        tunnel: w367 -> [w395]
                        tunnel: w365 -> [w386]
                        tunnel: w364 -> [w394]
                        tunnel: w362 -> [w393]
                        tunnel: w357 -> [w384]
                        tunnel: [w391] -> w352
                        tunnel: [w378] -> w350
                        tunnel: [w379] -> w348
                        tunnel: [w376] -> w346
                        tunnel: [w379] -> w344
                        tunnel: [w379] -> w342
                        tunnel: [w379] -> w340
                        tunnel: [w379] -> w338
                        tunnel: [w378] -> w336
                        tunnel: [w377] -> w334
                        tunnel: [w376] -> w332
                        tunnel: [w375] -> w330
                        tunnel: ["F Clear Plot B"] -> w328
                        tunnel: ["F Clear Plot A"] -> w326
                        tunnel: [w372] -> w324
                        tunnel: [w371] -> w322
                        tunnel: [w370] -> w320
                        tunnel: [w369] -> w318
                        tunnel: [w368] -> w316
                        tunnel: w352 -> [w417]
                        tunnel: [w417] -> w351
                        tunnel: w350 -> [w416]
                        tunnel: [w416] -> w349
                        tunnel: w348 -> [w415]
                        tunnel: [w415] -> w347
                        tunnel: w346 -> [w414]
                        tunnel: [w414] -> w345
                        tunnel: w344 -> [w413]
                        tunnel: [w413] -> w343
                        tunnel: w342 -> [w412]
                        tunnel: [w412] -> w341
                        tunnel: w340 -> [w411]
                        tunnel: [w411] -> w339
                        tunnel: w338 -> [w410]
                        tunnel: [w410] -> w337
                        tunnel: w336 -> [w409]
                        tunnel: [w409] -> w335
                        tunnel: w334 -> [w408]
                        tunnel: [w408] -> w333
                        tunnel: w332 -> [w407]
                        tunnel: [w407] -> w331
                        tunnel: w330 -> [w406]
                        tunnel: [w406] -> w329
                        tunnel: w328 -> [w405]
                        tunnel: [w405] -> w327
                        tunnel: w326 -> [w404]
                        tunnel: [w404] -> w325
                        tunnel: w324 -> [w403]
                        tunnel: [w403] -> w323
                        tunnel: w322 -> [w402]
                        tunnel: [w402] -> w321
                        tunnel: w320 -> [w401]
                        tunnel: [w401] -> w319
                        tunnel: w318 -> [w400]
                        tunnel: [w400] -> w317
                        tunnel: w316 -> [w399]
                        tunnel: [w399] -> w315
                        tunnel: w351 -> [w421]
                        tunnel: w349 -> [w455]
                        tunnel: w347 -> [w454]
                        tunnel: w345 -> [w453]
                        tunnel: w343 -> [w452]
                        tunnel: w341 -> [w450]
                        tunnel: w339 -> [w448]
                        tunnel: w337 -> [w446]
                        tunnel: w335 -> [w443]
                        tunnel: w333 -> [w442]
                        tunnel: w331 -> [w439]
                        tunnel: w329 -> [w438]
                        tunnel: w354 -> [w436]
                        tunnel: w327 -> [w435]
                        tunnel: w353 -> [w433]
                        tunnel: w325 -> [w432]
                        tunnel: w323 -> [w428]
                        tunnel: w321 -> [w427]
                        tunnel: w319 -> [w426]
                        tunnel: w317 -> [w423]
                        tunnel: w315 -> [w422]
                        tunnel: [w421] -> w314
                        tunnel: [w441] -> w313
                        tunnel: [w455] -> w312
                        tunnel: [w454] -> w311
                        tunnel: [w419] -> w310
                        tunnel: [w420] -> w309
                        tunnel: [w444] -> w308
                        tunnel: [w440] -> w307
                        tunnel: [w437] -> w306
                        tunnel: [w453] -> w305
                        tunnel: [w425] -> w304
                        tunnel: [w457] -> w355
                        tunnel: [w458] -> w356
                        tunnel: [w459] -> w358
                        tunnel: [w460] -> w359
                        tunnel: [w461] -> w360
                        tunnel: [w462] -> _
                        tunnel: [w463] -> w361
                        tunnel: [w464] -> w363
                        tunnel: [w465] -> w303
                        tunnel: [w466] -> w366
                        tunnel: [w467] -> _
                        tunnel: w314 -> [w467]
                        tunnel: w313 -> [w466]
                        tunnel: w312 -> [w465]
                        tunnel: w311 -> [w464]
                        tunnel: w310 -> [w463]
                        tunnel: w309 -> [w462]
                        tunnel: w308 -> [w461]
                        tunnel: w307 -> [w460]
                        tunnel: w306 -> [w459]
                        tunnel: w305 -> [w458]
                        tunnel: w304 -> [w457]
                        frame #0 {
                          w371 = u8 1 items=["Channel A", "Channel B"] ("Channel A/B for Parameter1")
                          w368 = u8 0 items=["Channel A", "Channel B"] ("Channel A/B for Parameter1")
                          n74 = Format Into String(0) -> (error out=w392:errorcluster)  [unwired: 3 in, 1 out]
                          n75 = Format Into String(0) -> (error out=w387:errorcluster)  [unwired: 3 in, 1 out]
                          n76 = call <instrlib>:"OE1022D_Read 1 parameter_mean.vi"("错误输入（无错误）"=w392, "Parameter"="Parameter A 2", "Channel (0: A)"=w368, "VISA resource name"=w386) -> ("error out"=w369:errorcluster, "Measurement"=w381:dbl, "VISA resource name out"=w391:refnum<visa-resource-name>)  [unwired: 5 in]
                          n77 = call <instrlib>:"OE1022D_Read 1 parameter_mean.vi"("Parameter 2"="Parameter B 2", "错误输入（无错误）"=w387, "Channel (0: A)"=w371, "VISA resource name"=w386) -> ("error out"=w372:errorcluster, "Measurement"=w380:dbl, "VISA resource name out"=w370:refnum<visa-resource-name>)  [unwired: 5 in]
                          n78 = Multiply(x=w381, y=1000.0) -> (x*y=w378:dbl)
                          "para1 Measurement (mV) 2" <- w378
                          n79 = Multiply(x=w380, y=1000000.0) -> (x*y=w376:dbl)
                          "para2 Measurement (uV) 2" <- w376
                          n80 = Build Array(w378) -> (w396:dbl[])
                          n81 = Build Array(w376) -> (w388:dbl[])
                          n82 = Select(t=w396, s="F Clear Plot A", f=w395) -> (s? t:f=w377:dbl[])
                          n83 = Select(t=w388, s="F Clear Plot B", f=w384) -> (s? t:f=w375:dbl[])
                          n84 = Build Array (concatenate)(w394, w393) -> (w379:dbl[])
                        }
                        frame #1 {
                          n85 = Wait (ms)(milliseconds to wait=u32 50) -> ()  [unwired: 1 out]
                        }
                        frame #2 {
                          n86 = Build Array (concatenate)(w443, w442) -> (w441:dbl[])
                          n87 = Build Array (concatenate)(w439, w438) -> (w437:dbl[])
                          n88 = Bundle(w448, w441) -> (→"RA-F":cluster{dbl[], dbl[]})  [unwired: 1 in]
                          n89 = Bundle(w450, w437) -> (→"Rh1B-F":cluster{dbl[], dbl[]})  [unwired: 1 in]
                          n90 = call <instrlib>:"OE1022D_Read 1 parameter_mean.vi"("错误输入（无错误）"=w423, "Parameter"="Phase A 2", "Channel (0: A)"=w422, "VISA resource name"=w421) -> ("error out"=w420:errorcluster, "Measurement"=w419:dbl)  [unwired: 5 in, 1 out]
                          "phase A 2" <- w419
                          n91 = call <instrlib>:"OE1022D_Read 1 parameter_mean.vi"("Parameter 2"="Phase B 2", "错误输入（无错误）"=w428, "Channel (0: A)"=w427, "VISA resource name"=w426) -> ("Measurement"=w425:dbl)  [unwired: 5 in, 2 out]
                          "phase B 2" <- w425
                          n92 = Build Array(w419) -> (w429:dbl[])
                          n93 = Build Array(w425) -> (w430:dbl[])
                          n94 = Select(t=w429, s=w432, f=w433) -> (s? t:f=w431:dbl[])
                          n95 = Select(t=w430, s=w435, f=w436) -> (s? t:f=w434:dbl[])
                          n96 = Build Array (concatenate)(w419, w431) -> (w444:dbl[])
                          n97 = Build Array (concatenate)(w425, w434) -> (w440:dbl[])
                          n98 = Bundle(w446, w444) -> (→"PhaseA-F":cluster{dbl[], dbl[]})  [unwired: 1 in]
                          n99 = Bundle(w452, w440) -> (→"Phaseh1B-F":cluster{dbl[], dbl[]})  [unwired: 1 in]
                        }
                        frame #3 {
                          n100 = Wait (ms)(milliseconds to wait=u32 50) -> ()  [unwired: 1 out]
                        }
                      }
                    }
                  }
                  n101 = case shown="True" w196 {
                    tunnel: w200 -> [_ w229]
                    tunnel: w201 -> [_ w234]
                    tunnel: w202 -> [_ w232]
                    tunnel: w199 -> [_ w228]
                    tunnel: w197 -> [_ w227]
                    tunnel: w198 -> [_ w226]
                    frame False {
                    }
                    frame True {
                      n102 = Build Array(w234, w229, w228, w227, w226) -> (w231:dbl[])
                      n103 = call-poly <vilib>:"Write Delimited Spreadsheet.vi"("file path (dialog if empty)"=w232, "format (%.3f)"="%.10f", "1D data"=w231, "append to file? (new file:F)"=TRUE) -> ()  [unwired: 10 in, 2 out]
                    }
                  }
                }
              }
            }
            frame True {
              n104 = Format Into String(format string="%.0f", "Set FIxed F (Oe)") -> (resulting string=w479:string)  [unwired: 2 in, 1 out]
              n105 = call "SetField.vi"("Mode"="Fixed F mode", "Approach"="Fixed Field Approach", "Rate"="FIxed F Rate (Oe/s)", "Field"="Set FIxed F (Oe)", "error in (no error)"=w490, "Instrument Ref In"=w491) -> ("error out"=w486:errorcluster, "Instrument Ref Out"=w488:refnum<k24>)  [unwired: 1 in, 1 out]
              n106 = Format Into String(initial string=w480, "Sweep", w477, w479, w476, w475) -> (resulting string=w482:string)  [unwired: 2 in, 1 out]
              n107 = local read "Delay(T/F)"() -> (w468:dbl)
              n108 = call "WaitFor.vi"("Delay"=w468, "Wait For Field"=TRUE, "error in (no error)"=w486, "Instrument Ref In"=w488) -> ("error out"=w487:errorcluster, "Instrument Ref Out"=w489:refnum<k24>)  [unwired: 6 in]
              n109 = String To Path(string=w482) -> (path=w481:path)
              n110 = for {
                N: w495 -> [_]
                tunnel: w496 -> [w525]
                tunnel: "Low Value (K)" -> [w519]
                tunnel: "High Value (K)" -> [w509]
                tunnel: w481 -> [w518]
                shift-right: [w514] -> _
                shift-left: _ -> [w513]
                shift-right: [w508] -> _
                shift-left: _ -> [w507]
                shift-right: [w506] -> _
                shift-left: _ -> [w505]
                shift-right: [w504] -> _
                shift-left: _ -> [w503]
                tunnel: w489 -> [w502]
                tunnel: w487 -> [w501]
                tunnel: w472 -> [w500]
                tunnel: [w499] -> w471
                tunnel: [w498] -> w470
                tunnel: w469 -> [w497]
                i -> [w511]
                n111 = Subtract(x=w509, y=w519) -> (x-y=w521:dbl)
                n112 = Add(x=1, y=w511) -> (x+y=→"T loop run":i32)
                n113 = Divide(x="Step(K)", y=1) -> (x/y=w520:dbl)
                n114 = Divide(x=w521, y=w520) -> (x/y=w517:dbl)
                n115 = Multiply(x=2, y=w517) -> (x*y=w516:dbl)
                n116 = Increment(x=w516) -> (x+1=w515:dbl)
                n117 = for {
                  N: w515 -> [_]
                  tunnel: w525 -> [w556]
                  tunnel: w520 -> [w552]
                  shift-right: [w543] -> w514
                  shift-left: w513 -> [w555]
                  tunnel: w517 -> [w550]
                  tunnel: w519 -> [w553]
                  tunnel: w509 -> [w551]
                  tunnel: w518 -> [w528]
                  shift-right: [w533] -> _
                  shift-left: _ -> [w546]
                  shift-right: [w545] -> w508
                  shift-left: w507 -> [w544]
                  shift-right: [w542] -> w506
                  shift-left: w505 -> [w541]
                  shift-right: [w540] -> w504
                  shift-left: w503 -> [w539]
                  tunnel: w502 -> [w538]
                  tunnel: w501 -> [w537]
                  tunnel: w500 -> [w536]
                  tunnel: [w535] -> w499
                  tunnel: [w534] -> w498
                  tunnel: w497 -> [w526]
                  i -> [w549]
                  n118 = Less Or Equal?(x=w549, y=w550) -> (x <= y?=w554:bool)
                  n119 = case shown="False" w554 {
                    tunnel: w553 -> [w566 w594]
                    tunnel: w549 -> [w575 w593]
                    tunnel: w552 -> [w574 w592]
                    tunnel: [w572 w590] -> w548
                    tunnel: w551 -> [w573 _]
                    tunnel: w550 -> [w568 _]
                    tunnel: w549 -> [w571 _]
                    frame False {
                      n120 = Multiply(x=w568, y=2) -> (x*y=w567:dbl)
                      n121 = Less Or Equal?(x=w571, y=w567) -> (x <= y?=w569:bool)
                      n122 = case shown="False" w569 {
                        tunnel: w575 -> [w582 w589]
                        tunnel: w574 -> [w580 w587]
                        tunnel: w573 -> [_ w585]
                        tunnel: [w578 w584] -> w572
                        tunnel: w568 -> [_ w583]
                        tunnel: w567 -> [w577 _]
                        tunnel: w566 -> [w576 _]
                        frame False {
                          n123 = Subtract(x=w582, y=w577) -> (x-y=w581:dbl)
                          n124 = Multiply(x=w580, y=w581) -> (x*y=w579:dbl)
                          n125 = Add(x=w576, y=w579) -> (x+y=w578:dbl)
                        }
                        frame True {
                          n126 = Subtract(x=w589, y=w583) -> (x-y=w588:dbl)
                          n127 = Multiply(x=w587, y=w588) -> (x*y=w586:dbl)
                          n128 = Subtract(x=w585, y=w586) -> (x-y=w584:dbl)
                        }
                      }
                    }
                    frame True {
                      n129 = Multiply(x=w592, y=w593) -> (x*y=w591:dbl)
                      n130 = Add(x=w594, y=w591) -> (x+y=w590:dbl)
                    }
                  }
                  n131 = Absolute Value(x=w548) -> (abs(x)=w547:dbl)
                  n132 = stacked-sequence {
                    tunnel: w556 -> [_ _ w695]
                    tunnel: w547 -> [w613 _ w633]
                    tunnel: w555 -> [_ _ w697]
                    tunnel: [_ _ w696] -> w543
                    tunnel: [_ _ w694] -> w529
                    tunnel: [_ _ w693] -> w533
                    tunnel: w546 -> [_ _ w692]
                    tunnel: [_ _ w691] -> w530
                    tunnel: [_ _ w690] -> w545
                    tunnel: w544 -> [_ _ w684]
                    tunnel: [_ _ w689] -> w542
                    tunnel: w541 -> [_ _ w685]
                    tunnel: [_ _ w688] -> w540
                    tunnel: w539 -> [_ _ w687]
                    tunnel: [_ _ w634] -> w531
                    tunnel: [_ _ w686] -> w532
                    tunnel: w538 -> [w612 _ _]
                    tunnel: w537 -> [w611 _ _]
                    tunnel: w536 -> [_ w630 _]
                    tunnel: [w597 _ _] -> w535
                    tunnel: [w596 _ _] -> w534
                    tunnel: [_ _ w633] -> w527
                    frame #0 {
                      n133 = call "SetTemperature.vi"("Approach"="Sweep Temperature Approach", "Rate"="Sweep T  Rate (K/min)", "Temperature"=w613, "error in (no error)"=w611, "Instrument Ref In"=w612) -> ("error out"=w609:errorcluster, "Instrument Ref Out"=w610:refnum<k24>)  [unwired: 2 in, 1 out]
                      n134 = local read "Delay(T/F)"() -> (w595:dbl)
                      n135 = call "WaitFor.vi"("Delay"=w595, "Wait For Temperature"=TRUE ("WaitForTemperature"), "error in (no error)"=w609, "Instrument Ref In"=w610) -> ("error out"=w600:errorcluster, "Instrument Ref Out"=w599:refnum<k24>)  [unwired: 6 in]
                      n136 = for {
                        N: 20 -> [_]
                        shift-right: [w629] -> _
                        shift-left: TRUE -> [w627]
                        shift-right: [w624] -> w597
                        shift-left: w600 -> [w626]
                        tunnel: w599 -> [w623]
                        tunnel: [w621] -> w596
                        tunnel: [w618] -> w606
                        tunnel: [w617] -> w605
                        tunnel: [w619] -> w603 mode=indexing
                        tunnel: [w620] -> w604 mode=indexing
                        n137 = local write "Measuring T"(w627) -> ()
                        n138 = Not(x=w627) -> (.not. x?=w629:bool)
                        n139 = call "GetTemperature.vi"("error in (no error)"=w626, "Instrument Ref In"=w623) -> ("Temperature\nStatus"=w617:i32, "Temperature"=w620:dbl, "error out"=w625:errorcluster, "Instrument Ref Out"=w622:refnum<k24>)  [unwired: 3 in, 1 out]
                        n140 = Wait (ms)(milliseconds to wait=u32 200) -> ()  [unwired: 1 out]
                        n141 = call "GetField.vi"("error in (no error)"=w625, "Instrument Ref In"=w622) -> ("Field\nStatus"=w618:i32, "Field"=w619:dbl, "error out"=w624:errorcluster, "Instrument Ref Out"=w621:refnum<k24>)  [unwired: 3 in, 1 out]
                      }
                      "Field Status" <- w606
                      "Temperature Status" <- w605
                      n142 = call-poly <vilib>:"Mean.vi"("X"=w603) -> ("mean"=→"Fixed Field":dbl)  [unwired: 1 out]
                      n143 = call-poly <vilib>:"Mean.vi"("X"=w604) -> ("mean"=→"Measured Temperature":dbl)  [unwired: 1 out]
                      "Temperature Setting" <- w613
                      "Measuring T" <- FALSE
                    }
                    frame #1 {
                      n144 = Multiply(x=w630, y=1000) -> (x*y=w632:dbl)
                      n145 = Wait (ms)(milliseconds to wait=w632) -> ()  [unwired: 1 out]
                    }
                    frame #2 {
                      n146 = flat-sequence {
                        tunnel: w697 -> [w725]
                        tunnel: w695 -> [w716]
                        tunnel: w633 -> [w724]
                        tunnel: w692 -> [w723]
                        tunnel: w687 -> [w714]
                        tunnel: [w721] -> w683
                        tunnel: [w708] -> w681
                        tunnel: [w709] -> w679
                        tunnel: [w706] -> w677
                        tunnel: [w709] -> w675
                        tunnel: [w709] -> w673
                        tunnel: [w709] -> w671
                        tunnel: [w709] -> w669
                        tunnel: [w708] -> w667
                        tunnel: [w707] -> w665
                        tunnel: [w706] -> w663
                        tunnel: [w705] -> w661
                        tunnel: ["T Clear Plot B"] -> w659
                        tunnel: ["T Clear Plot A"] -> w657
                        tunnel: [w702] -> w655
                        tunnel: [w701] -> w653
                        tunnel: [w700] -> w651
                        tunnel: [w699] -> w649
                        tunnel: [w698] -> w647
                        tunnel: w683 -> [w747]
                        tunnel: [w747] -> w682
                        tunnel: w681 -> [w746]
                        tunnel: [w746] -> w680
                        tunnel: w679 -> [w745]
                        tunnel: [w745] -> w678
                        tunnel: w677 -> [w744]
                        tunnel: [w744] -> w676
                        tunnel: w675 -> [w743]
                        tunnel: [w743] -> w674
                        tunnel: w673 -> [w742]
                        tunnel: [w742] -> w672
                        tunnel: w671 -> [w741]
                        tunnel: [w741] -> w670
                        tunnel: w669 -> [w740]
                        tunnel: [w740] -> w668
                        tunnel: w667 -> [w739]
                        tunnel: [w739] -> w666
                        tunnel: w665 -> [w738]
                        tunnel: [w738] -> w664
                        tunnel: w663 -> [w737]
                        tunnel: [w737] -> w662
                        tunnel: w661 -> [w736]
                        tunnel: [w736] -> w660
                        tunnel: w659 -> [w735]
                        tunnel: [w735] -> w658
                        tunnel: w657 -> [w734]
                        tunnel: [w734] -> w656
                        tunnel: w655 -> [w733]
                        tunnel: [w733] -> w654
                        tunnel: w653 -> [w732]
                        tunnel: [w732] -> w652
                        tunnel: w651 -> [w731]
                        tunnel: [w731] -> w650
                        tunnel: w649 -> [w730]
                        tunnel: [w730] -> w648
                        tunnel: w647 -> [w729]
                        tunnel: [w729] -> w646
                        tunnel: w682 -> [w751]
                        tunnel: w680 -> [w785]
                        tunnel: w678 -> [w784]
                        tunnel: w676 -> [w783]
                        tunnel: w674 -> [w782]
                        tunnel: w672 -> [w780]
                        tunnel: w670 -> [w778]
                        tunnel: w668 -> [w776]
                        tunnel: w666 -> [w773]
                        tunnel: w664 -> [w772]
                        tunnel: w662 -> [w769]
                        tunnel: w660 -> [w768]
                        tunnel: w685 -> [w766]
                        tunnel: w658 -> [w765]
                        tunnel: w684 -> [w763]
                        tunnel: w656 -> [w762]
                        tunnel: w654 -> [w758]
                        tunnel: w652 -> [w757]
                        tunnel: w650 -> [w756]
                        tunnel: w648 -> [w753]
                        tunnel: w646 -> [w752]
                        tunnel: [w751] -> w645
                        tunnel: [w771] -> w644
                        tunnel: [w785] -> w643
                        tunnel: [w784] -> w642
                        tunnel: [w749] -> w641
                        tunnel: [w750] -> w640
                        tunnel: [w774] -> w639
                        tunnel: [w770] -> w638
                        tunnel: [w767] -> w637
                        tunnel: [w783] -> w636
                        tunnel: [w755] -> w635
                        tunnel: [w789] -> w686
                        tunnel: [w790] -> w634
                        tunnel: [w787] -> w688
                        tunnel: [w791] -> w689
                        tunnel: [w792] -> w690
                        tunnel: [w793] -> _
                        tunnel: [w794] -> w691
                        tunnel: [w795] -> w693
                        tunnel: [w796] -> w694
                        tunnel: [w786] -> w696
                        tunnel: [w797] -> _
                        tunnel: w645 -> [w797]
                        tunnel: w644 -> [w786]
                        tunnel: w643 -> [w796]
                        tunnel: w642 -> [w795]
                        tunnel: w641 -> [w794]
                        tunnel: w640 -> [w793]
                        tunnel: w639 -> [w792]
                        tunnel: w638 -> [w791]
                        tunnel: w637 -> [w787]
                        tunnel: w636 -> [w790]
                        tunnel: w635 -> [w789]
                        frame #0 {
                          w701 = u8 1 items=["Channel A", "Channel B"] ("Channel A/B for Parameter1")
                          w698 = u8 0 items=["Channel A", "Channel B"] ("Channel A/B for Parameter1")
                          n147 = Format Into String(0) -> (error out=w722:errorcluster)  [unwired: 3 in, 1 out]
                          n148 = Format Into String(0) -> (error out=w717:errorcluster)  [unwired: 3 in, 1 out]
                          n149 = call <instrlib>:"OE1022D_Read 1 parameter_mean.vi"("错误输入（无错误）"=w722, "Parameter"="Parameter A", "Channel (0: A)"=w698, "VISA resource name"=w716) -> ("error out"=w699:errorcluster, "Measurement"=w711:dbl, "VISA resource name out"=w721:refnum<visa-resource-name>)  [unwired: 5 in]
                          n150 = call <instrlib>:"OE1022D_Read 1 parameter_mean.vi"("Parameter 2"="Parameter B", "错误输入（无错误）"=w717, "Channel (0: A)"=w701, "VISA resource name"=w716) -> ("error out"=w702:errorcluster, "Measurement"=w710:dbl, "VISA resource name out"=w700:refnum<visa-resource-name>)  [unwired: 5 in]
                          n151 = Multiply(x=w711, y=1000.0) -> (x*y=w708:dbl)
                          "para1 Measurement (mV)" <- w708
                          n152 = Multiply(x=w710, y=1000000.0) -> (x*y=w706:dbl)
                          "para2 Measurement (uV)" <- w706
                          n153 = Build Array(w708) -> (w726:dbl[])
                          n154 = Build Array(w706) -> (w718:dbl[])
                          n155 = Select(t=w726, s="T Clear Plot A", f=w725) -> (s? t:f=w707:dbl[])
                          n156 = Select(t=w718, s="T Clear Plot B", f=w714) -> (s? t:f=w705:dbl[])
                          n157 = Build Array (concatenate)(w724, w723) -> (w709:dbl[])
                        }
                        frame #1 {
                          n158 = Wait (ms)(milliseconds to wait=u32 50) -> ()  [unwired: 1 out]
                        }
                        frame #2 {
                          n159 = Build Array (concatenate)(w773, w772) -> (w771:dbl[])
                          n160 = Build Array (concatenate)(w769, w768) -> (w767:dbl[])
                          n161 = Bundle(w778, w771) -> (→"RA-T":cluster{dbl[], dbl[]})  [unwired: 1 in]
                          n162 = Bundle(w780, w767) -> (→"Rh1B-T":cluster{dbl[], dbl[]})  [unwired: 1 in]
                          n163 = call <instrlib>:"OE1022D_Read 1 parameter_mean.vi"("错误输入（无错误）"=w753, "Parameter"="Phase A", "Channel (0: A)"=w752, "VISA resource name"=w751) -> ("error out"=w750:errorcluster, "Measurement"=w749:dbl)  [unwired: 5 in, 1 out]
                          "phase A" <- w749
                          n164 = call <instrlib>:"OE1022D_Read 1 parameter_mean.vi"("Parameter 2"="Phase B", "错误输入（无错误）"=w758, "Channel (0: A)"=w757, "VISA resource name"=w756) -> ("Measurement"=w755:dbl)  [unwired: 5 in, 2 out]
                          "phase B" <- w755
                          n165 = Build Array(w749) -> (w759:dbl[])
                          n166 = Build Array(w755) -> (w760:dbl[])
                          n167 = Select(t=w759, s=w762, f=w763) -> (s? t:f=w761:dbl[])
                          n168 = Select(t=w760, s=w765, f=w766) -> (s? t:f=w764:dbl[])
                          n169 = Build Array (concatenate)(w749, w761) -> (w774:dbl[])
                          n170 = Build Array (concatenate)(w755, w764) -> (w770:dbl[])
                          n171 = Bundle(w776, w774) -> (→"PhaseA-T":cluster{dbl[], dbl[]})  [unwired: 1 in]
                          n172 = Bundle(w782, w770) -> (→"Phaseh1-T":cluster{dbl[], dbl[]})  [unwired: 1 in]
                        }
                        frame #3 {
                          n173 = Wait (ms)(milliseconds to wait=u32 50) -> ()  [unwired: 1 out]
                        }
                      }
                    }
                  }
                  n174 = case shown="True" w526 {
                    tunnel: w529 -> [_ w560]
                    tunnel: w527 -> [_ w565]
                    tunnel: w528 -> [_ w563]
                    tunnel: w530 -> [_ w559]
                    tunnel: w531 -> [_ w558]
                    tunnel: w532 -> [_ w557]
                    frame False {
                    }
                    frame True {
                      n175 = Build Array(w565, w560, w559, w558, w557) -> (w562:dbl[])
                      n176 = call-poly <vilib>:"Write Delimited Spreadsheet.vi"("file path (dialog if empty)"=w563, "format (%.3f)"="%.10f", "1D data"=w562, "append to file? (new file:F)"=TRUE) -> ()  [unwired: 10 in, 2 out]
                    }
                  }
                }
              }
            }
          }
        }
      }
    }
    frame #2 {
      n177 = case shown="True" "Initialize" {
        tunnel: w800 -> [w801 w804]
        tunnel: w799 -> [w802 w803]
        frame False {
          n178 = Close Reference(reference=w802, error in (no error)=w801) -> ()  [unwired: 1 out]
        }
        frame True {
          w810 = 0 items=["Linear", "NoOvershoot", "Oscillate"] ("Approach")
          w811 = 0 items=["Persistent", "Driven"] ("Mode")
          w807 = 0 items=["FastSettle", "NoOvershoot"] ("Approach")
          n179 = call "SetTemperature.vi"("Approach"=w807, "Rate"=20.0, "Temperature"=120.0, "error in (no error)"=w804, "Instrument Ref In"=w803) -> ("error out"=w815:errorcluster, "Instrument Ref Out"=w814:refnum<k24>)  [unwired: 2 in, 1 out]
          n180 = call "SetField.vi"("Mode"=w811, "Approach"=w810, "Rate"=200.0, "Field"=0.0, "error in (no error)"=w815, "Instrument Ref In"=w814) -> ("error out"=w812:errorcluster, "Instrument Ref Out"=w813:refnum<k24>)  [unwired: 1 in, 1 out]
          n181 = Close Reference(reference=w813, error in (no error)=w812) -> ()  [unwired: 1 out]
        }
      }
    }
  }
  n182 = while {
    tunnel: w3 -> [w818]
    tunnel: w2 -> [w817]
    stop <- "?" stop-if-true
    n183 = for {
      N: 10 -> [_]
      shift-right: [w833] -> _
      shift-left: w817 -> [w835]
      tunnel: w818 -> [w832]
      tunnel: [w830] -> _
      tunnel: [w827] -> w824
      tunnel: [w826] -> w823
      tunnel: [w828] -> w821 mode=indexing
      tunnel: [w829] -> w822 mode=indexing
      n184 = call "GetTemperature.vi"("error in (no error)"=w835, "Instrument Ref In"=w832) -> ("Temperature\nStatus"=w826:i32, "Temperature"=w829:dbl, "error out"=w834:errorcluster, "Instrument Ref Out"=w831:refnum<k24>)  [unwired: 3 in, 1 out]
      n185 = Wait (ms)(milliseconds to wait=u32 200) -> ()  [unwired: 1 out]
      n186 = call "GetField.vi"("error in (no error)"=w834, "Instrument Ref In"=w831) -> ("Field\nStatus"=w827:i32, "Field"=w828:dbl, "error out"=w833:errorcluster, "Instrument Ref Out"=w830:refnum<k24>)  [unwired: 3 in, 1 out]
    }
    "Field Status" <- w824
    "Temperature Status" <- w823
    n187 = call-poly <vilib>:"Mean.vi"("X"=w821) -> ("mean"=→"Field":dbl)  [unwired: 1 out]
    n188 = call-poly <vilib>:"Mean.vi"("X"=w822) -> ("mean"=→"Temperature":dbl)  [unwired: 1 out]
  }
